vi "Glbl Stop.vi"() -> ()   [LabVIEW 2017]
panel:
  in  "Glbl Stop":bool
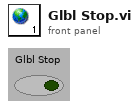
[diagram p1: front panel]
diagram:
